vi "Time Flatten.vi"() -> ()   [LabVIEW 2017]
panel:
  in  "Numeric 2":i32
  in  "Boolean":bool
  in  "Numeric":i32
  out "x-y":u32
  # "50% faster to do byte stuff than flatten to string"
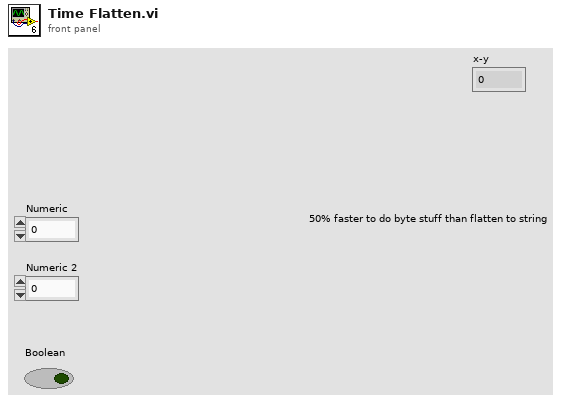
[diagram p1: front panel]
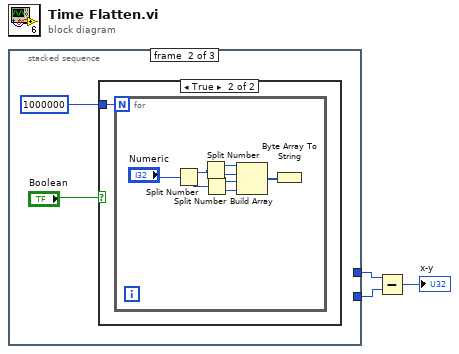
[diagram p0: block diagram]
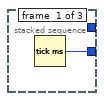
[diagram p2: hidden frame]
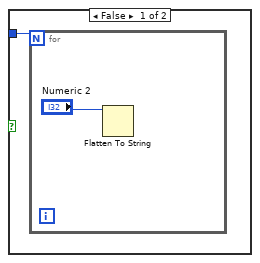
[diagram p3: hidden frame]
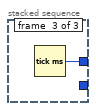
[diagram p4: hidden frame]
diagram:
  n1 = stacked-sequence {
    tunnel: [w4 _ _] -> w2
    tunnel: [_ _ w18] -> w3
    frame #0 {
      n2 = Tick Count (ms)() -> (millisecond timer value=w4:u32)
    }
    frame #1 {
      n3 = case shown="True" "Boolean" {
        tunnel: 1000000 -> [w7 w9]
        frame False {
          n4 = for {
            N: w7 -> [_]
            n5 = Flatten To String(anything="Numeric 2") -> ()  [unwired: 3 in, 3 out]
          }
        }
        frame True {
          n6 = for {
            N: w9 -> [_]
            n7 = Split Number(x="Numeric") -> (hi(x)=w15:u16, lo(x)=w16:u16)
            n8 = Split Number(x=w15) -> (hi(x)=w14:u8, lo(x)=w13:u8)
            n9 = Split Number(x=w16) -> (hi(x)=w12:u8, lo(x)=w11:u8)
            n10 = Build Array(w14, w13, w12, w11) -> (w10:u8[])
            n11 = Byte Array To String(unsigned byte array=w10) -> ()  [unwired: 1 out]
          }
        }
      }
    }
    frame #2 {
      n12 = Tick Count (ms)() -> (millisecond timer value=w18:u32)
    }
  }
  n13 = Subtract(x=w3, y=w2) -> (x-y=→"x-y":u32)
